vi "Read Dev Span.vi"(8 "error in (no error)":errorcluster, 11 "VISA resource name":refnum<visa-resource-name>) -> (0 "error out":errorcluster, 2 "dev span":cluster{"dev span cap":dbl, "dev span loss":dbl}, 3 "VISA resource name out":refnum<visa-resource-name>)   [LabVIEW 2019, in "Andeen-Hagerling 2700A.lvlib"]
doc: "Returns the distance between the upper and lower bounds of the\ninput deviation capacitance and loss spans in pF and jpF\nrespectively. These deviation spans correspond directly to the\nanalog output voltage spans for capacitance and loss respectively."
uses:
  Andeen-Hagerling 2700A.lvlib
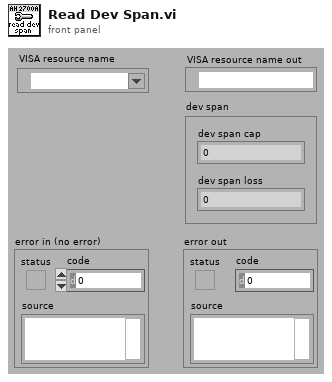
[diagram p1: front panel]
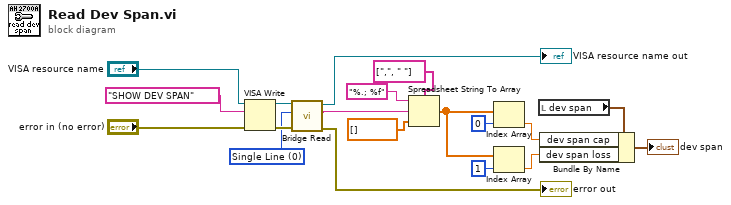
[diagram p0: block diagram]
diagram:
  w1 = u16 0 items=["Single Line", "Multi-Line"] ("Multiline")
  n1 = VISA Write(VISA resource name="VISA resource name", write buffer="SHOW DEV SPAN" ("command"), error in (no error)="error in (no error)") -> (VISA resource name out=w6:refnum<visa-resource-name>, error out=w5:errorcluster)  [unwired: 1 out]
  n2 = call "Bridge Read.vi"("error in (no error)"=w5, "multiline"=w1, "VISA resource name"=w6) -> ("error out"=→"error out":errorcluster, "read buffer"=w3:string, "VISA resource name out"=→"VISA resource name out":refnum<visa-resource-name>)  [unwired: 6 in]
  n3 = Spreadsheet String To Array(delimiter (Tab)=string[] [",", " "], format string="%.; %f", spreadsheet string=w3, array type (2D Dbl)=dbl[] []) -> (array=w12:dbl[])
  n4 = Index Array(array=w12, index=0) -> (element=w9:dbl)
  n5 = Index Array(array=w12, index=1) -> (element=w8:dbl)
  n6 = local read "dev span"() -> (w10:cluster{"dev span cap":dbl, "dev span loss":dbl})
  n7 = Bundle By Name(cluster=w10, "dev span cap"=w9, "dev span loss"=w8) -> (→"dev span":cluster{"dev span cap":dbl, "dev span loss":dbl})
